vi "Dashboard Main.vi"() -> ()   [LabVIEW 2017]
uses:
  RoboRio Code/Systems/Autonomous/Autonomous/ENUM_Auto_AutoMode.ctl
  RoboRio Code/Systems/Arm/ENUM_SM_State.ctl
  RoboRio Code/Systems/Claw Rotation/ENUM_SM_State.ctl
  RoboRio Code/Systems/Lift/ENUM_SM_State.ctl
  <vilib>/Utility/miscctls.llb/LVRowAndColumnTypeDef.ctl
  <vilib>/event_ctls.llb/eventvkey.ctl
  RoboRio Code/TypeDef/CLUSTER_Sensitivities.ctl
  <vilib>/Rock Robotics/Network Tables/NT Read Numeric Array.vi
  <vilib>/Rock Robotics/WPI/Dashboard/WPI_DashboardLogging Global.vi
  RoboRio Code/Systems/Arm/Arm.lvlib
  RoboRio Code/Systems/Claw Rotation/Claw_Rotation.lvlib
  RoboRio Code/Systems/Lift/Lift.lvlib
panel:
  in  "Camera Settings Right":T1={"Frame Rate"=30, "Compression"=30, "Size"=1, "DB Camera Config"=FALSE} {"Frame Rate" scale=1.0..30.0; "Compression" scale=100.0..-1.0; "Size" items=["640x480", "320x240", "160x120"]}
  in  "Camera Name Right":string(combo)="No Camera Selection"
  out "Camera Info":cluster{"Mbps LED":bool, "Mbps":dbl, "fps":dbl} {"fps" format="%#.1g"; "Mbps" format="%#.1g"}
  in  "Camera Settings":T1={"Frame Rate"=30, "Compression"=30, "Size"=1, "DB Camera Config"=FALSE} {"Frame Rate" scale=1.0..30.0; "Compression" scale=100.0..-1.0; "Size" items=["640x480", "320x240", "160x120"]}
  in  "TCP":refnum<k5>
  in  "Rec Mode":enum32{"Stop", "Record", "Playback"}(radio)
  out "Robot IP":string
  out "Image Message":string="Timeout in Camera Communications"
  in  "Dashboard Tab":T2(tab)
  in  "Select Auto":string(combo)="Select Autonomous ..."
  out "NT Connection":bool
  out "MotorChart R":cluster{"Numeric":dbl, "Numeric":dbl}(graph)
  out "MotorChart L":cluster{"Numeric":dbl, "Numeric":dbl}(graph)
  out "MotorSliders R":cluster{"MotorSlide1":dbl, "MotorSlide2":dbl} {"MotorSlide2" scale=-1.0..1.0 scale format="%#_2e"; "MotorSlide1" scale=-1.0..1.0 scale format="%#_2e"}
  out "MotorSliders L":cluster{"MotorSlide1":dbl, "MotorSlide2":dbl} {"MotorSlide2" scale=-1.0..1.0 scale format="%#_2e"; "MotorSlide1" scale=-1.0..1.0 scale format="%#_2e"}
  out "Gyro":dbl(knob) scale=0.0..360.0
  out "JS1 Z":dbl(slide) scale=-1.0..1.0 scale format="%#_2e"
  out "JS1 Graph":cluster{"X":dbl, "Y":dbl}[](graph)
  out "JS1 Buttons":T3
  out "JS2 Z":dbl(slide) scale=-1.0..1.0 scale format="%#_2e"
  out "JS2 Graph":cluster{"X":dbl, "Y":dbl}[](graph)
  out "JS2 Buttons":T3
  out "Mode":T4(ring)=enum."Auto Disabled"
  out "Camera Image Right":T5(plugin-control)
  out "Lift State":T6
  out "Claw Rotation State":T7
  out "Arm State":T8
  in  "Low Gear Sen Min":dbl
  in  "Low Gear Sen Max":dbl
  in  "High Gear Sen Min":dbl
  in  "High Gear Sen Max":dbl
  out "Bottom Arm":bool
  out "Top Arm":bool
  out "Bottom Claw":bool
  out "Top Claw":bool
  out "Bottom Lift":bool
  out "Top Lift":bool
  out "Cube":bool
  out "Road Nav":bool
  out "Cube":bool
  out "Low Gear":bool
  out "High Gear":bool
  out "Drive Mode":T9(ring)
  out "Lock Angle":bool
  out "Turbo Enabled":bool
  out "Comp. Running":bool
  out "Comp. Enabled":bool
  in  "Reset Max RPM":bool
  out "Right Max":dbl
  out "Left Max":dbl
  out "Right":dbl
  out "Left":dbl
  out "Battery Meter":dbl(knob) scale=0.0..15.0
  in  "Cube Steer Scale":dbl
  in  "Cube Deadband":dbl
  in  "Auto Route":T10
  out "V Min":dbl
  out "V Max":dbl
  in  "V Values":cluster{dbl, dbl}(slide) scale=0.0..255.0
  out "S Min":dbl
  out "S Max":dbl
  in  "S Values":cluster{dbl, dbl}(slide) scale=0.0..255.0
  out "H Min":dbl
  out "H Max":dbl
  in  "H Values":cluster{dbl, dbl}(slide) scale=0.0..255.0
  in  "Test Slider":dbl(slide) scale=0.0..100.0 scale format="%#_3g"
  in  "On/Off":bool caption="Solenoid"
  in  "Test Name":u16(ring) items=["Select the test to run..."]
  in  "Test Tree":string(tree)
  in  "Motor":cluster{"Value":dbl, "Enable":bool} {"Value" scale=-1.0..1.0 scale format="%#_3g"}
  out "Progress":T11 {"Test Progress" scale=0.0..100.0}
  in  "Rev/Fwd":cluster{"Forward":bool, "Reverse":bool}
  in  "Test Ring":u16(ring) items=["Monochrome", "Color"]
  out "Cmd Status":string
  in  "Execute Command":bool
  in  "Command Params":string[][](table)
  in  "Command Selection":i32(listbox)
  in  "CheckList":i32(listbox)
  out "Tree":string(tree)
  out "Manipulator Mietus":picture
  out "Handsome Hale":picture
  out "Jeffery Junior":picture
  out "Camera Image":T5(plugin-control)
  in  "Camera Name":string(combo)="No Camera Selection"
  # "HW"
  # "HW"
  # "Joysticks"
  # "Drive Motors"
  # "Front"
  # "Right"
  # "Left"
  # "Back"
  # "Drive RPMs"
  # "Limit Switches"
  # "Drive"
  # "Object Tracker"
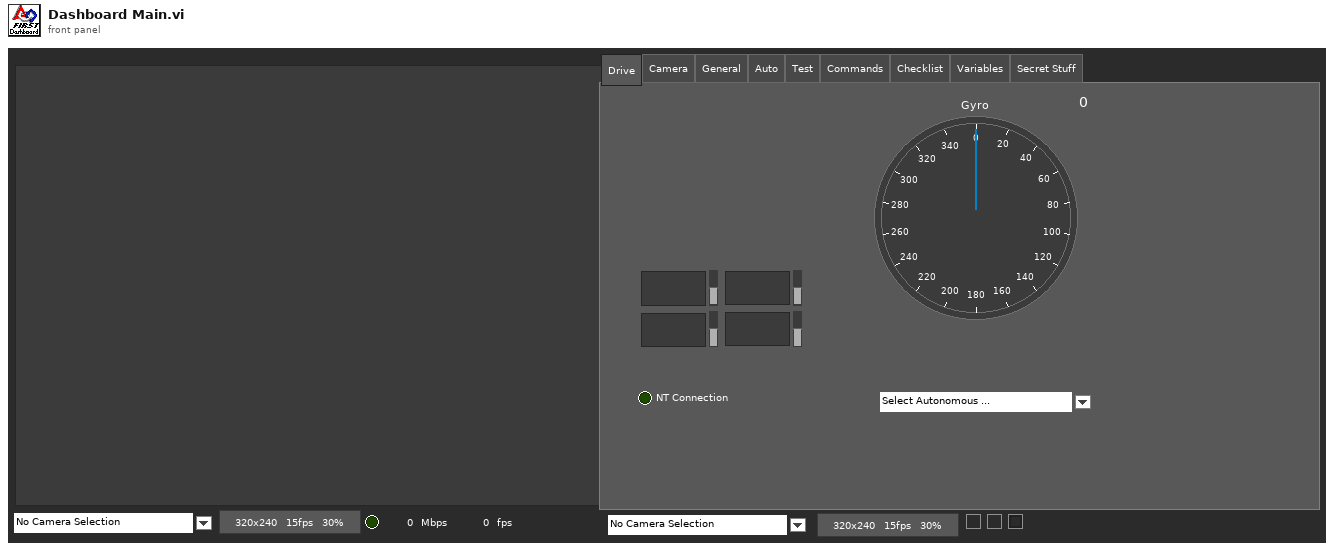
[diagram p1: front panel]
types:
  T1 = cluster{"Frame Rate":i32, "Compression":i32, "Size":u16, "DB Camera Config":bool}
  T2 = enum32{"Drive", "Camera", "General", "Auto", "Test", "Commands", "Checklist", "Variables", "Secret Stuff"}
  T3 = cluster{bool, bool, bool, bool, bool, bool, bool, bool, bool, bool, bool, bool}
  T4 = enum8{"Tele-Op Disabled", "Tele-Op Enabled", "Auto Disabled", "Auto Enabled", "Test Disabled", "Test Enabled", "Disconnected", "No Code", "E-Stop"}
  T5 = typedef "IMAQ Image.ctl" = refnum<image>
  T6 = typedef "Lift.lvlib/ENUM_SM_State.ctl" = enum16{"Startup", "Idle", "F_Manual", "Manual", "Position - Moving", "Position - Holding", "Shutdown"}
  T7 = typedef "Claw_Rotation.lvlib/ENUM_SM_State.ctl" = enum16{"Startup", "Idle", "F_Manual", "Manual", "Position - Moving", "Position - Holding", "Shutdown"}
  T8 = typedef "Arm.lvlib/ENUM_SM_State.ctl" = enum16{"Startup", "Idle", "F_Manual", "Manual", "Position - Moving", "Position - Holding", "Shutdown"}
  T9 = enum16{"Motion Profile", "CrossLineAuto", "VBus", "Stop"}
  T10 = typedef "ENUM_Auto_AutoMode.ctl" = enum16{"No Movement", "Scale And Switch", "Switch", "Scale", "Cross Line"}
  T11 = cluster{"Test Progress":u8, "Test Progress Text":string}
  T12 = cluster{"Save Path":path, "Interval (s)":dbl, "Keep":i32}
  T13 = enum32{"General", "Drive", "Camera", "Basic", "Custom", "Test", "Commands", "Checklist", "Variables"}
  T14 = typedef "Image Type" = u32
  T15 = cluster{"IDs":cluster{"RPC field ID":u16, "Unique ID":u16}, "String":string}
  T16 = enum32{"Drive", "Camera", "General", "Auto", "Test", "Commands", "Checklist", "Variables"}
  T17 = cluster{"Camera Image":refnum<vi>, "Dashboard Tab":refnum<vi>, void, "Rec Mode":refnum<vi>, "Test Slider":refnum<vi>, "On/Off ":refnum<vi>, "Test Ring":refnum<vi>, "Rev/Fwd":refnum<vi>, "Test Name":refnum<vi>, "Motor":refnum<vi>, "Progress":refnum<vi>, "CheckList":refnum<vi>, "Tree":refnum<vi>, "Test Tree":refnum<vi>, "Command Params":refnum<vi>, "Command Selection":refnum<vi>, "Execute Command":refnum<vi>, "Cmd Status":refnum<vi>, "Camera Settings":refnum<vi>, "Camera Name":refnum<vi>, "Camera Info":refnum<vi>, "Camera Settings Right":refnum<vi>, "Camera Name Right":refnum<vi>, "Camera Image Right":refnum<vi>}
  T18 = cluster{"Camera Name":string, string, "Saved DB Images Info":cluster{"Save Path":path, "Interval (s)":dbl, "Keep":i32}}
  T19 = cluster{"Camera Name Right":string, string, "Saved DB Images Info":cluster{"Save Path":path, "Interval (s)":dbl, "Keep":i32}}
  T20 = typedef "CLUSTER_Sensitivities.ctl" = cluster{"High Gear Max":dbl, "High Gear Min":dbl, "Low Gear Max":dbl, "Low Gear Min":dbl}
  T21 = cluster{"Error Strings":string, "Disable Counts":cluster{u16, u16}, "Rail Faults":cluster{u16, u16, u16}, "Robot IP":string, "DB Mode":u8, "Event Info":cluster{"Name":string, "Type":u8, "Number":u16, "Replay":u8}}
  T22 = cluster{"Storage":cluster{"Disk Free":u64, "RAM Block":u32, "RAM free":u32}, "CPU Utilization":cluster{"CPU % ISR":sgl, "CPU % Time Crit":sgl, "CPU % Timed Str":sgl, "CPU % High":sgl, "CPU % Above":sgl, "CPU % Normal":sgl, "CPU % Low":sgl}, "CAN":cluster{"% Bus Utilization":sgl, "Bus Off Cnt":u32, "TX_FIFO Full Cnt":u32, "Receive Error Cnt":u8, "Transmit Error Cnt":u8}, "HID":cluster{"HID Outputs":u32, "Rumble Low":u16, "Rumble High":u16}[]}
  T23 = cluster{"Status bits":cluster{"Test Mode":bool, "Autonomous":bool, "Enabled":bool, "Code Start":bool, "Brownout":bool, "Reserved 2":bool, "Reserved 3":bool, "E-Stop":bool}, "Code Trace":cluster{"Disabled":bool, "TeleOp":bool, "Auto":bool, "Test":bool}, "Controller Type":enum16{"unknown", "cRIO", "roboRio"}, "Code?":enum16{"unknown", "noCode", "code"}, "Battery V":dbl}
  T24 = cluster{"Control Bits":cluster{"TestMode":bool, "Autonomous":bool, "Enabled":bool, "FMS Present":bool, bool, bool, bool, "E-Stop":bool}, "Team Station ":u8, "Countdown":sgl, "Joystick Values":cluster{"Axes":dbl[], "Buttons":bool[], "POVs":i16[]}[]}
  T25 = cluster{"Axes":dbl[], "Buttons":bool[], "POVs":i16[]}[]
  T26 = typedef "Cluster_Compressor.ctl" = cluster{"Compressor Running":bool, "Compressor Enabled":bool}
  T27 = typedef "CLUSTER_CMD_WC_Drive.ctl" = cluster{"Drive_Mode":T28, "VBus":T29, "Profile":T31, "Zero Drive Encoders":bool, "Set Target Position(IN)":dbl, "Target Angle(Degree)":dbl, "Lock Angle":bool, "Zero YAW":bool, "Follow Cubes":bool, "Follow Road":bool}
  T28 = typedef "ENUM_WC_Drive_DriveMode.ctl" = enum16{"Motion Profile", "CrossLineAuto", "VBus", "Stop"}
  T29 = typedef "CLUSTER_Drive_ACT Loop_VBus Data.ctl" = cluster{"Drive":T30, "Turbo":bool}
  T30 = typedef "CLUSTER_X and Y.ctl" = cluster{"Steer":dbl, "Throtle":dbl}
  T31 = typedef "CLUSTER_Drive_ACT Loop_Profile Data.ctl" = cluster{"Start":bool}
  T32 = cluster{"Axes":dbl[], "Buttons":bool[], "POVs":i16[]}
  T33 = cluster{"Buttons[0]":bool, "Buttons[1]":bool, "Buttons[2]":bool, "Buttons[3]":bool, "Buttons[4]":bool, "Buttons[5]":bool, "Buttons[6]":bool, "Buttons[7]":bool, "Buttons[8]":bool, "Buttons[9]":bool, "Buttons[10]":bool, "Buttons[11]":bool}
  T34 = typedef "CLUSTER_Limit_Switches.ctl" = cluster{"Cube":bool, "Top Arm":bool, "Bottom Claw":bool, "Top Lift":bool, "Bottom Arm":bool, "Bottom Lift":bool, "Top Claw":bool}
  T35 = cluster{"Operation":enum16{"Update", "Clear"}, "Color Box":u32}[]
  T36 = typedef "eventvkey.ctl" = enum16{"ASCII", "Enter", "Return", "Shift", "Ctrl", "Alt", "Cmd", "Opt", "Caps", "NumLock", "Clear", "Break", "Up", "Down", "Left", "Right", "Insert", "Delete", "Home", "End", "PageUp", "PageDown", "Escape", "Help", "Pause", "ScrollLock", "F1", "F2", "F3", "F4", "F5", "F6", "F7", "F8", "F9", "F10", "F11", "F12", "F13", "F14", "F15", "F16", "F17", "F18", "F19", "F20", "F21", "F22", "F23", "F24", "Play", "VolumeUp", "VolumeDown", "Mute", "Two Byte Char"}
  T37 = cluster{"Image Size":bool, "Image Type":bool, "Pixel Value":bool, "ROI Information":bool, "Zoom Factor":bool}
  T38 = cluster{"Operation":enum16{"Update", "Clear"}, "Color Box":u32}
  T39 = typedef "LVRowAndColumnTypeDef.ctl" = cluster{"Row":i32, "Column":i32}
  T40 = cluster{"Shift":bool, "Ctrl":bool, "Alt":bool, "Cmd":bool, "Opt":bool}
  T41 = typedef "imagedata.ctl" = cluster{"image type":i32, "image depth":i32, "image":u8[], "mask":u8[], "colors":u32[], "Rectangle":cluster{"left":i16, "top":i16, "right":i16, "bottom":i16}}
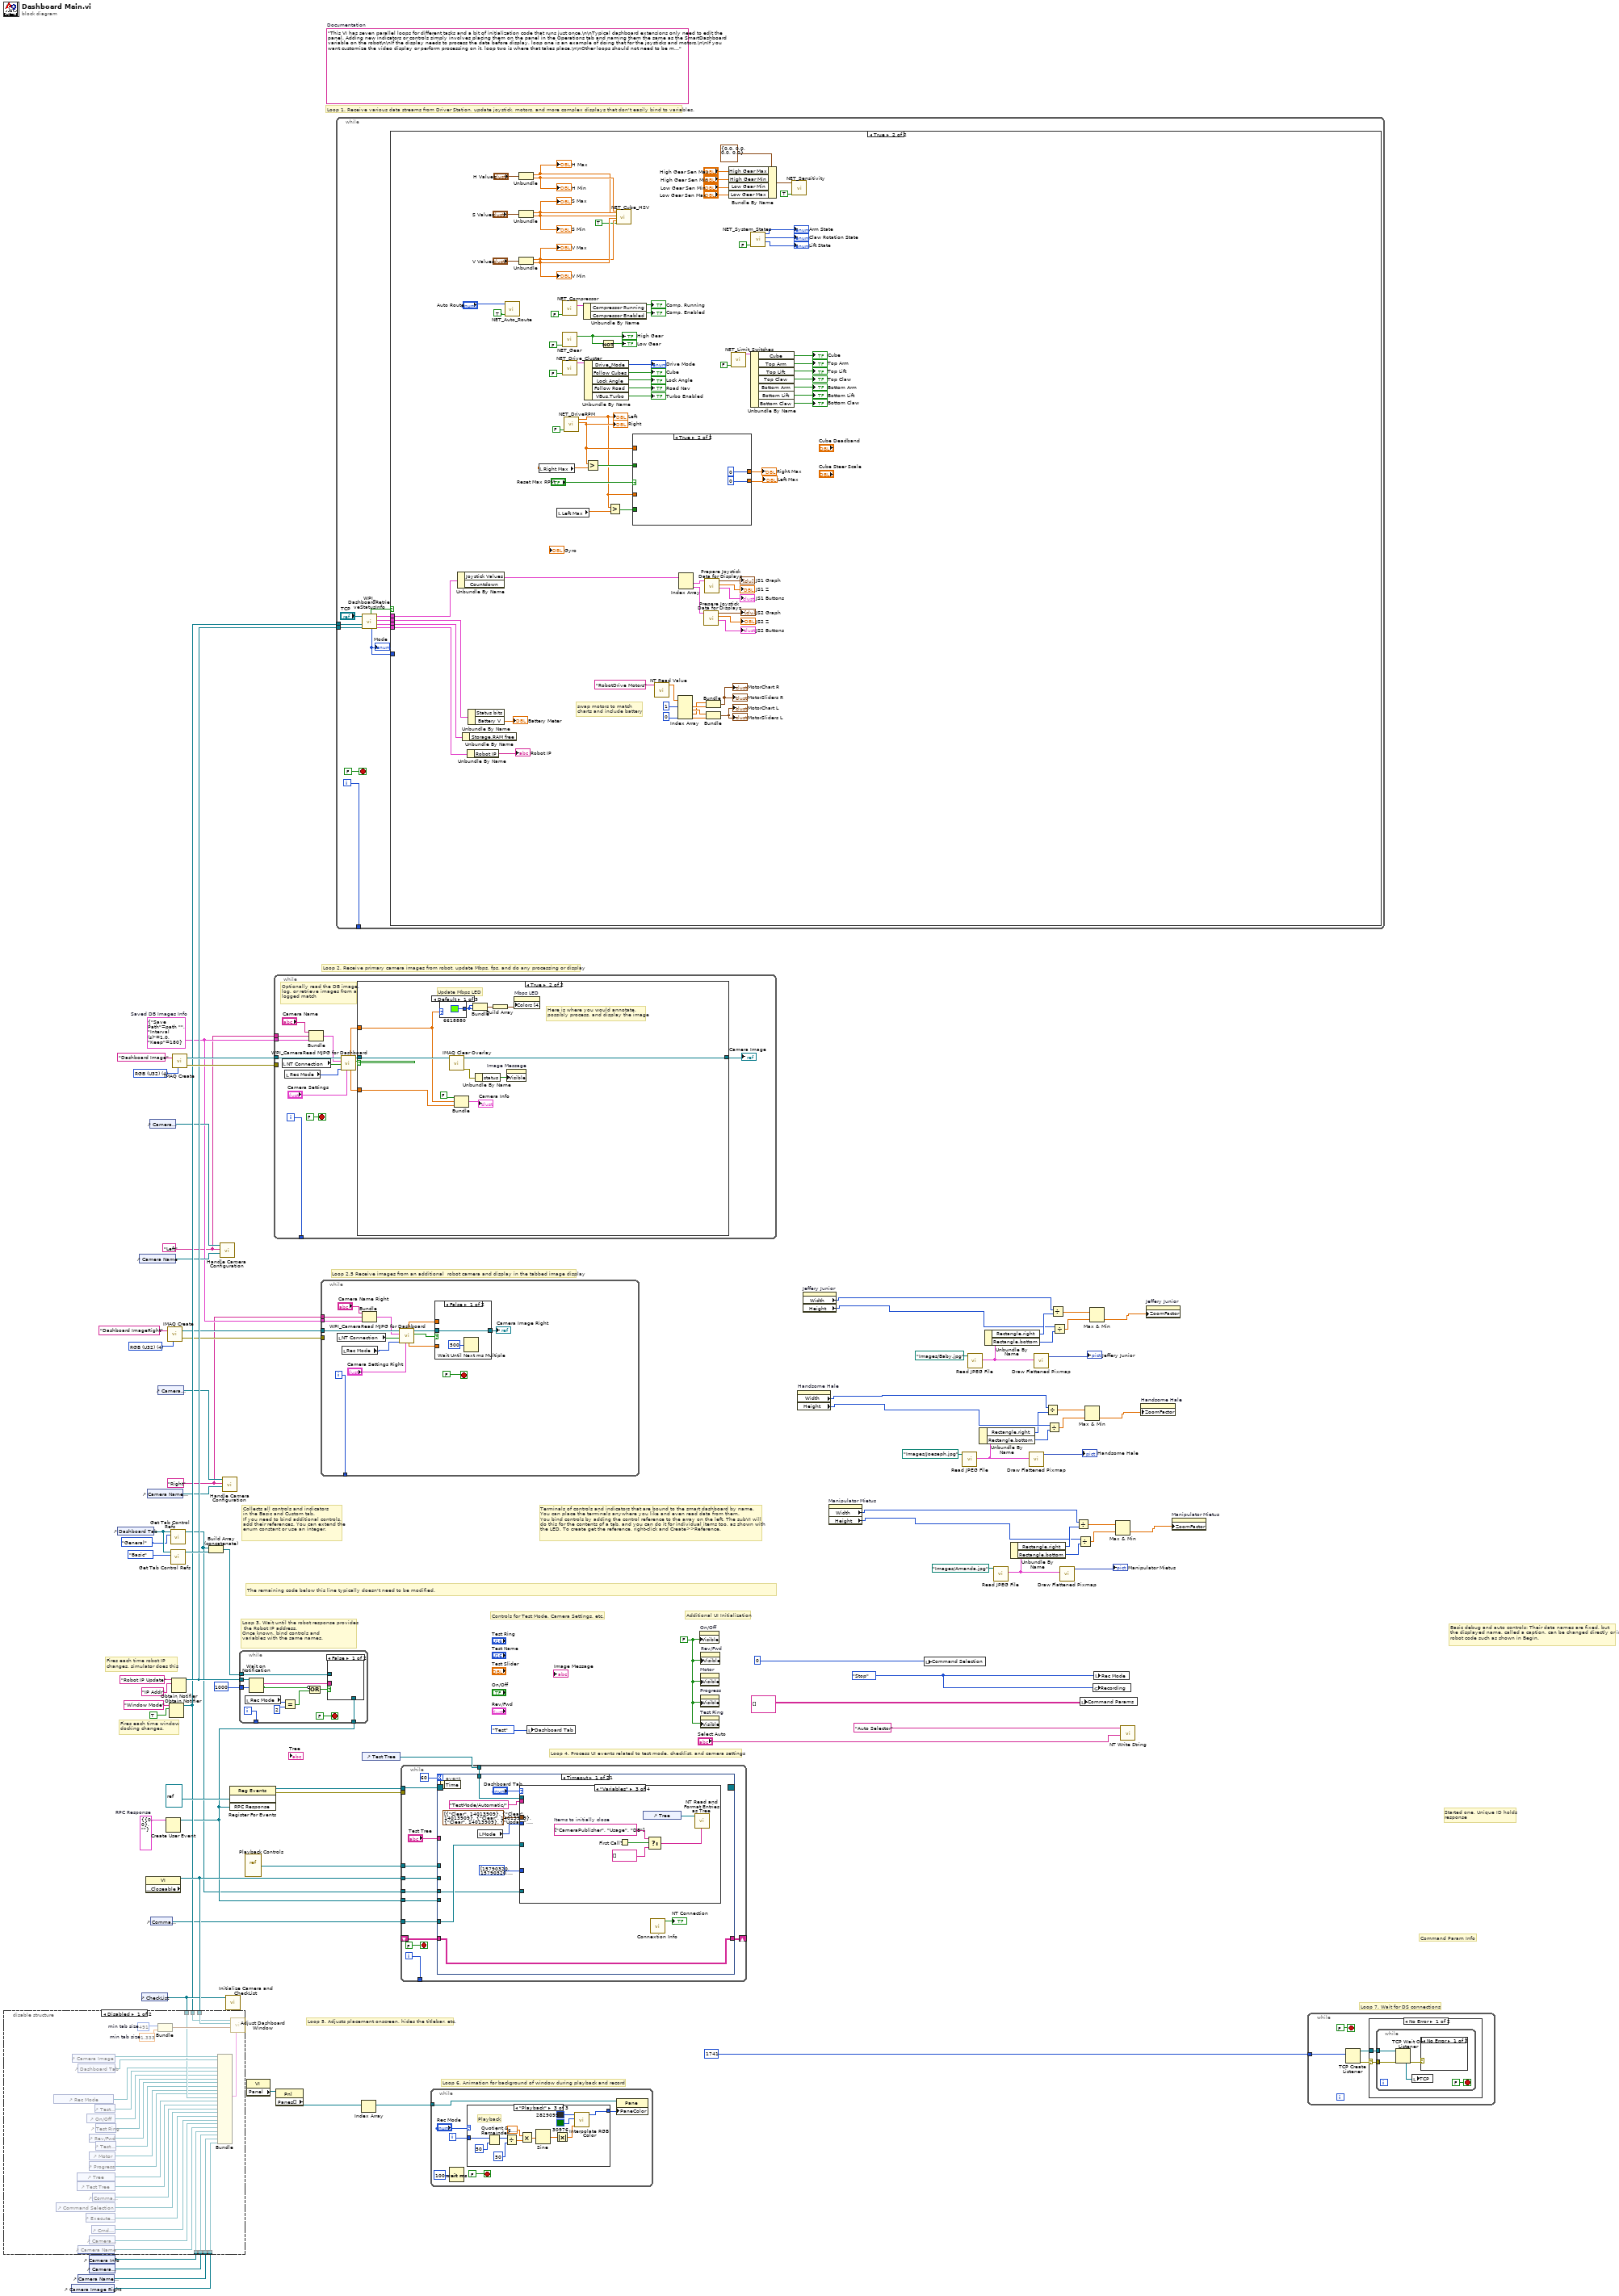
[diagram p0: block diagram]
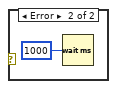
[diagram p4: hidden frame]
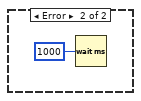
[diagram p5: hidden frame]
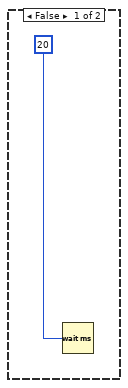
[diagram p6: hidden frame]
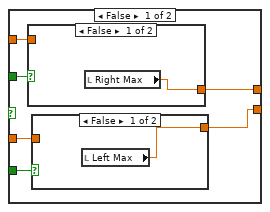
[diagram p7: hidden frame]
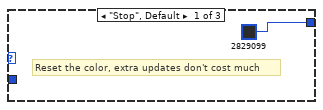
[diagram p10: hidden frame]
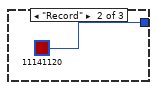
[diagram p11: hidden frame]
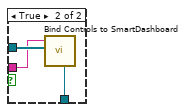
[diagram p12: hidden frame]
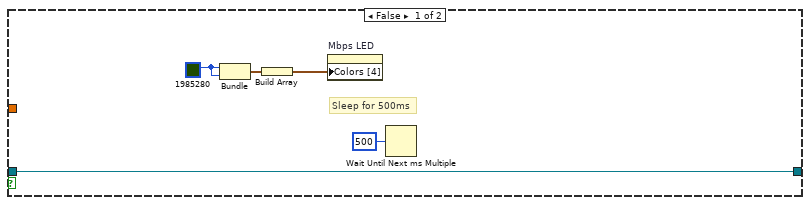
[diagram p13: hidden frame]
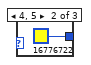
[diagram p14: hidden frame]
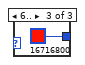
[diagram p15: hidden frame]
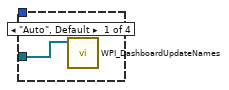
[diagram p16: hidden frame]
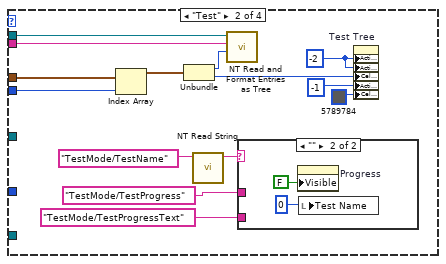
[diagram p17: hidden frame]
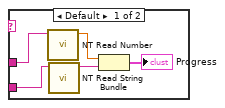
[diagram p18: hidden frame]
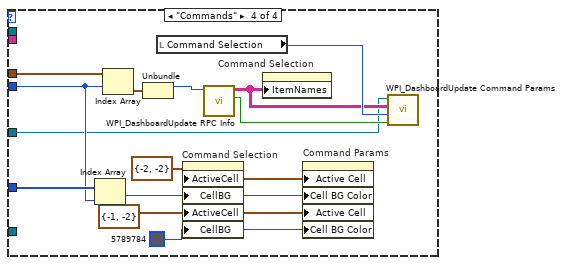
[diagram p19: hidden frame]
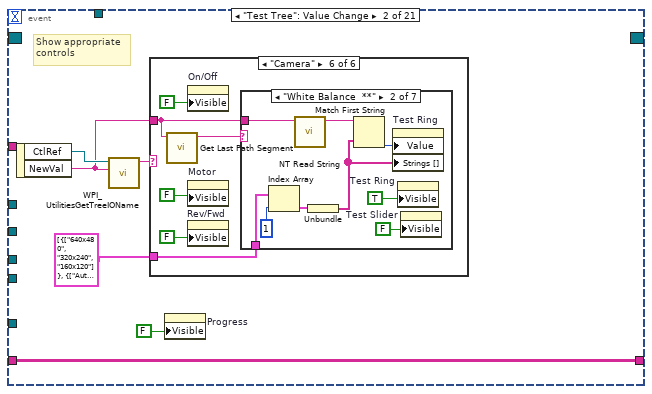
[diagram p20: hidden frame]
diagram:
  w34 = T12 {"Save Path"=path "", "Interval (s)"=1.0, "Keep"=180}  # Saved DB Images Info
  w33 = "Right"
  w32 = "Left"
  w44 = T14 4 items=["Grayscale (U8)", "Grayscale (I16)", "Grayscale (SGL)", "Complex (CSG)", "RGB (U32)", "HSL (U32)", "RGB (U64)"] ("Image Type")
  w55 = T15 {"IDs"={"RPC field ID"=0, "Unique ID"=0}, "String"=""}  # RPC Response
  w66 = enum32{"Stop", "Record", "Playback"}."Stop" ("Rec Mode")
  w60 = FALSE ("Visible")
  (unwired) "This VI has seven parallel loops for different tasks and a bit of initialization code that runs just once.\n\nTypical dashboard extensions only need to edit the panel. Adding new indicators or controls simply involves placing them on the panel in the Operations tab and naming them the same as the SmartDashboard variable on the robot\n\nIf the display needs to process the data before display, loop one is an example of doing that for the joysticks and motors.\n\nIf you want customize the video display or perform processing on it, loop two is where that takes place.\n\nOther loops should not need to be modified. They are pretty standard, and document the task they perform."  # Documentation
  w83 = T14 4 items=["Grayscale (U8)", "Grayscale (I16)", "Grayscale (SGL)", "Complex (CSG)", "RGB (U32)", "HSL (U32)", "RGB (U64)"] ("Image Type")
  # "Loop 2.5 Receive images from an additional  robot camera and display in the tabbed image display"
  # "Command Param Info"
  # "Started one, Unique ID holds\nresponse"
  # "Loop 7. Wait for DS connections"
  # "Basic debug and auto controls: Their data names are fixed, but\nthe displayed name, called a caption, can be changed directly or in\nrobot code such as shown in Begin."
  # "Controls for Test Mode, Camera Settings, etc."
  # "Additional UI Initialization"
  # "Loop 6. Animation for background of window during playback and record"
  # "Fires each time robot IP\nchanges, simulator does this"
  # "Fires each time window\ndocking changes."
  # "Collects all controls and indicators\nin the Basic and Custom tab.\nIf you need to bind additional controls,\nadd their references. You can extend the\nenum constant or use an integer."
  # "The remaining code below this line typically doesn't need to be modified."
  # "Loop 4. Process UI events related to test mode, checklist, and camera settings"
  # "Terminals of controls and indicators that are bound to the smart dashboard by name.\nYou can place the terminals anywhere you like and even read data from them.\nYou bind controls by adding the control reference to the array on the left. The subVI will\ndo this for the contents of a tab, and you can do it for individual items too, as shown with\nthe LED. To create get the reference, right-click and Create>>Reference."
  # "Loop 3. Wait until the robot response provides\n the Robot IP address.\nOnce known, bind controls and\nvariables with the same names."
  # "Loop 5. Adjusts placement onscreen, hides the titlebar, etc."
  # "Loop 1. Receive various data streams from Driver Station, update joystick, motors, and more complex displays that don't easily bind to variables."
  # "Loop 2. Receive primary camera images from robot, update Mbps, fps, and do any processing or display"
  n1 = control-ref of="Camera Image Right"() -> (w37:refnum<vi>)
  n2 = control-ref of="Camera Name Right"() -> (w38:refnum<vi>)
  n3 = control-ref of="Camera Info"() -> (w49:refnum<vi>)
  n4 = control-ref of="Camera Settings Right"() -> (w39:refnum<vi>)
  n5 = control-ref of="Dashboard Tab"() -> (w64:refnum<vi>)
  n6 = control-ref of="Camera Name"() -> (w50:refnum<vi>)
  n7 = control-ref of="CheckList"() -> (w61:refnum<vi>)
  n8 = property class="VI" props=["Front Panel.Closeable"]() -> (reference out=w65:refnum<vi>)  [unwired: 2 in, 2 out]
  n9 = control-ref of="Camera Name Right"() -> (w40:refnum<vi>)
  n10 = control-ref of="Camera Settings"() -> (w51:refnum<vi>)
  n11 = control-ref of="Command Params"() -> (w52:refnum<vi>)
  n12 = control-ref of="Camera Settings Right"() -> (w41:refnum<vi>)
  n13 = Create User Event(user event datatype=w55) -> (user event=w53:refnum<user-event>)  [unwired: 1 in, 1 out]
  n14 = call "IMAQ Create"("Image Name"="Dashboard ImageRight", "Image Type"=w44) -> ("New Image"=w43:T5, "error out"=w42:errorcluster)  [unwired: 2 in, 1 out]
  n15 = Obtain Notifier(name (unnamed)="Window Mode", notification data type=TRUE) -> (notifier out=w58:refnum<notifier>)  [unwired: 2 in, 2 out]
  n16 = disable-structure shown="Disabled" {
    disable-tunnel: w65 -> [w113 _]
    disable-tunnel: w61 -> [w105 _]
    disable-tunnel: w58 -> [w94 _]
    disable-tunnel: w49 -> [w87 _]
    disable-tunnel: w39 -> [w86 _]
    disable-tunnel: w38 -> [w85 _]
    disable-tunnel: w37 -> [w84 _]
    frame Disabled {
      w110 = 491  # min tab size
      w109 = 1.333  # min tab size
      n17 = control-ref of="Rec Mode"() -> (w100:refnum<vi>)
      n18 = control-ref of="Command Selection"() -> (w91:refnum<vi>)
      n19 = control-ref of="Camera Image"() -> (w112:refnum<vi>)
      n20 = control-ref of="Tree"() -> (w104:refnum<vi>)
      n21 = control-ref of="Test Tree"() -> (w103:refnum<vi>)
      n22 = control-ref of="Dashboard Tab"() -> (w111:refnum<vi>)
      n23 = control-ref of="Camera Name"() -> (w88:refnum<vi>)
      n24 = control-ref of="Execute Command"() -> (w92:refnum<vi>)
      n25 = control-ref of="On/Off"() -> (w98:refnum<vi>)
      n26 = control-ref of="Progress"() -> (w95:refnum<vi>)
      n27 = control-ref of="Camera Settings"() -> (w89:refnum<vi>)
      n28 = control-ref of="Rev/Fwd"() -> (w96:refnum<vi>)
      n29 = control-ref of="Motor"() -> (w101:refnum<vi>)
      n30 = control-ref of="Cmd Status"() -> (w90:refnum<vi>)
      n31 = control-ref of="Command Params"() -> (w93:refnum<vi>)
      n32 = control-ref of="Test Slider"() -> (w99:refnum<vi>)
      n33 = control-ref of="Test Ring"() -> (w97:refnum<vi>)
      n34 = control-ref of="Test Name"() -> (w102:refnum<vi>)
      n35 = Bundle("min tab size"=w110, "min tab size"=w109) -> (w108:cluster{"min tab size":i32, "min tab size":dbl})  [unwired: 1 in]
      n36 = Bundle("Camera Image"=w112, "Dashboard Tab"=w111, "Rec Mode"=w100, "Test Slider"=w99, "On/Off"=w98, "Test Ring"=w97, "Rev/Fwd"=w96, "Test Name"=w102, "Motor"=w101, "Progress"=w95, "CheckList"=w105, "Tree"=w104, "Test Tree"=w103, "Command Params"=w93, "Command Selection"=w91, "Execute Command"=w92, "Cmd Status"=w90, "Camera Settings"=w89, "Camera Name"=w88, "Camera Info"=w87, "Camera Settings Right"=w86, "Camera Name Right"=w85, "Camera Image Right"=w84) -> (w106:T17, w107)  [unwired: 1 in]
      n37 = call "Adjust Dashboard Window.vi"("Sizing Refnums"=w106, "Size Constraints"=w108, "VI"=w113, "WIn Mode"=w94) -> ()  [unwired: 8 in]
    }
    frame Enabled {
    }
  }
  n38 = call <vilib>:"Get Tab Control Refs.vi"("Page Index"=T13."General" ("Dashboard Tab"), "TabControl in"=w64) -> ("ControlsOnPage"=w48:refnum<vi>[])  [unwired: 9 in]
  n39 = call <vilib>:"Get Tab Control Refs.vi"("Page Index"=T13."Basic" ("Dashboard Tab"), "TabControl in"=w64) -> ("ControlsOnPage"=w63:refnum<vi>[])  [unwired: 9 in]
  n40 = Obtain Notifier(name (unnamed)="Robot IP Update", notification data type="IP Addr" ("name (unnamed)")) -> (notifier out=w59:refnum<notifier>)  [unwired: 2 in, 2 out]
  n41 = call "IMAQ Create"("Image Name"="Dashboard Image", "Image Type"=w83) -> ("New Image"=w81:T5, "error out"=w80:errorcluster)  [unwired: 2 in, 1 out]
  n42 = Build Array (concatenate)(w48, w63) -> (w62:refnum<vi>[])
  n43 = call "Handle Camera Configuration.vi"("CameraNameRef"=w50, "Display Name"=w32, "ClusterRef"=w51) -> ()  [unwired: 9 in]
  n44 = call "Handle Camera Configuration.vi"("CameraNameRef"=w40, "Display Name"=w33, "ClusterRef"=w41) -> ()  [unwired: 9 in]
  n45 = call "Initialize Camera and CheckList.vi"("ListBox in"=w61) -> ()  [unwired: 11 in]
  n46 = register-events(refnum<vi> refnum, w53) -> (reference out=w70:refnum<event-registration>, error out=w69:errorcluster)  [unwired: 2 in]
  n47 = while {
    tunnel: w62 -> [w125]
    tunnel: w59 -> [w123]
    tunnel: [w121] -> _
    tunnel: u32 1000 ("milliseconds to wait") -> [w120]
    tunnel: w53 -> [w114]
    i -> [w121]
    stop <- FALSE stop-if-true
    n48 = local read "Rec Mode"() -> (w116:enum32{"Stop", "Record", "Playback"})
    n49 = Wait on Notification(notifier=w123, timeout in ms (-1)=w120) -> (notification=w122:string, timed out?=w118:bool)  [unwired: 2 in, 2 out]
    n50 = Equal?(x=w116, y=u16 2 ("Rec Mode")) -> (x = y?=w117:bool)
    n51 = Compound Arithmetic op=OR(invert w118, w117) -> (w119:bool)
    n52 = case shown="False" w119 {
      tunnel: w125 -> [_ w128]
      tunnel: w122 -> [_ w127]
      tunnel: w114 -> [_ w126]
      frame False {
      }
      frame True {
        n53 = call <vilib>:"Bind Controls to SmartDashboard.vi"("RPC ref"=w126, "Bound Control Refs"=w128, "Server IP Address"=w127) -> ()  [unwired: 9 in]
      }
    }
  }
  n54 = vi-ref "Playback Controls.vi"() -> (w71:refnum<vi>)
  n55 = property class="VI"() -> ("Panel"=w73:refnum<vi>)  [unwired: 2 in, 2 out]
  n56 = while {
    tunnel: w81 -> [w141]
    tunnel: w80 -> [_]
    tunnel: [w142] -> _
    tunnel: w34 -> [w132]
    tunnel: w32 -> [w129]
    i -> [w142]
    stop <- FALSE stop-if-true
    # "Optionally read the DB image,\nlog, or retrieve images from a\nlogged match"
    n57 = local read "NT Connection"() -> (w133:bool)
    n58 = local read "Rec Mode"() -> (w137:enum32{"Stop", "Record", "Playback"})
    n59 = Bundle("Camera Name"="Camera Name", w129, "Saved DB Images Info"=w132) -> (w131:T18)  [unwired: 1 in]
    n60 = call <vilib>:"WPI_CameraRead MJPG for Dashboard.vi"("Camera Settings"="Camera Settings", "Rec Mode"=w137, "NT Connection"=w133, "Capture Info"=w131, "Refnum in"=w141) -> ("Active"=w139:bool, "Refnum out"=w140:T5, "FPS"=w138:dbl, "Bandwidth (Mbps)"=w136:dbl)  [unwired: 3 in]
    n61 = case shown="True" w139 {
      tunnel: w140 -> [w144 w155]
      tunnel: w136 -> [_ w152]
      tunnel: w138 -> [_ w153]
      tunnel: [w144 w149] -> w134
      frame False {
        w146 = u32 1985280 ("Color Box")
        # "Sleep for 500ms"
        n62 = Bundle("Color Box"=w146, "Color Box"=w146) -> (w147:cluster{"Color Box":u32, "Color Box":u32})  [unwired: 1 out]
        n63 = Build Array(w147) -> (w145:cluster{"Color Box":u32, "Color Box":u32}[])
        n64 = property on="Mbps LED" class="Bool (strict)"("Colors [4]"=w145) -> ()  [unwired: 2 in, 2 out]
        n65 = Wait Until Next ms Multiple(millisecond multiple=u32 500) -> ()  [unwired: 1 out]
      }
      frame True {
        # "Here is where you would annotate,\npossibly process, and display the image"
        # "Update Mbps LED"
        n66 = case shown="Default" w152 {
          tunnel: [u32 6618880 ("Color Box") u32 16776722 ("Color Box") u32 16716800 ("Color Box")] -> w156
          frame Default {
          }
          frame 4, 5 {
          }
          frame 6.. {
          }
        }
        n67 = call "IMAQ Clear Overlay"("Image"=w155) -> ("error out"=w158:errorcluster, "Image Out"=w149:T5)  [unwired: 2 in, 7 out]
        n68 = Bundle(FALSE, "Bandwidth (Mbps)"=w152, "FPS"=w153) -> (→"Camera Info":cluster{bool, "Bandwidth (Mbps)":dbl, "FPS":dbl})  [unwired: 1 in]
        n69 = Bundle("Color Box"=w156, "Color Box"=w156) -> (w157:cluster{"Color Box":u32, "Color Box":u32})  [unwired: 1 out]
        n70 = Unbundle By Name(w158) -> ("status"=w159:bool)
        n71 = Build Array(w157) -> (w154:cluster{"Color Box":u32, "Color Box":u32}[])
        n72 = property on="Image Message" class="Str"("Visible"=w159) -> ()  [unwired: 2 in, 2 out]
        n73 = property on="Mbps LED" class="Bool (strict)"("Colors [4]"=w154) -> ()  [unwired: 2 in, 2 out]
      }
    }
    "Camera Image" <- w134
  }
  n74 = property class="Pnl"(reference=w73) -> ("Panes[]"=w74:refnum<vi>[])  [unwired: 1 in, 2 out]
  n75 = while {
    tunnel: w43 -> [w177]
    tunnel: w42 -> [_]
    tunnel: [w172] -> _
    tunnel: w34 -> [w166]
    tunnel: w33 -> [w163]
    i -> [w172]
    stop <- FALSE stop-if-true
    n76 = local read "NT Connection"() -> (w167:bool)
    n77 = local read "Rec Mode"() -> (w176:enum32{"Stop", "Record", "Playback"})
    n78 = Bundle("Camera Name Right"="Camera Name Right", w163, "Saved DB Images Info"=w166) -> (w165:T19)  [unwired: 1 in]
    n79 = call <vilib>:"WPI_CameraRead MJPG for Dashboard.vi"("Camera Settings"="Camera Settings Right", "Rec Mode"=w176, "NT Connection"=w167, "Capture Info"=w165, "Refnum in"=w177) -> ("Active"=w171:bool, "Refnum out"=w174:T5, "FPS"=w169:dbl, "Bandwidth (Mbps)"=w170:dbl)  [unwired: 3 in]
    n80 = case shown="False" w171 {
      tunnel: w174 -> [w178 w180]
      tunnel: w170 -> [_ _]
      tunnel: w169 -> [_ _]
      tunnel: [w178 w180] -> w168
      frame False {
        n81 = Wait Until Next ms Multiple(millisecond multiple=u32 500) -> ()  [unwired: 1 out]
      }
      frame True {
      }
    }
    "Camera Image Right" <- w168
  }
  n82 = while {
    tunnel: [w190] -> _
    tunnel: w59 -> [w184]
    tunnel: w58 -> [w181]
    i -> [w190]
    stop <- FALSE stop-if-true
    n83 = call <vilib>:"WPI_DashboardRetrieveStatusInfo.vi"("Binding Refnum"=w184, "Window Mode Notifier"=w181, "TCP Cnx"="TCP") -> ("Power and Errors"=w185:T21, "Robot Metrics"=w188:T22, "Status Info"=w189:T23, "Control Info"=w186:T24, "Robot Mode"=w183:T4, "Process?"=w187:bool)  [unwired: 3 in]
    "Mode" <- w183
    n84 = case shown="True" w187 {
      tunnel: w189 -> [_ w273]
      tunnel: w188 -> [_ w272]
      tunnel: w186 -> [_ w271]
      tunnel: w185 -> [_ w270]
      tunnel: w183 -> [_ _]
      frame False {
        n85 = Wait (ms)(milliseconds to wait=u32 20) -> ()  [unwired: 1 out]
      }
      frame True {
        # "swap motors to match\ncharts and include battery"
        n86 = Unbundle By Name(w271) -> ("Joystick Values"=w261:T25)  [unwired: 1 out]
        n87 = Unbundle By Name(w272) -> ()  [unwired: 1 out]
        n88 = Unbundle By Name(w270) -> ("Robot IP"=→"Robot IP":string)
        n89 = Unbundle By Name(w273) -> ("Battery V"=→"Battery Meter":dbl)  [unwired: 1 out]
        n90 = call "NET_Auto_Route.vi"("Read(F) Write(T)"=TRUE, "Route In"="Auto Route") -> ()  [unwired: 9 in, 1 out]
        n91 = Unbundle("H Values") -> (w245:dbl, w246:dbl)
        "H Max" <- w245
        "H Min" <- w246
        n92 = Unbundle("S Values") -> (w243:dbl, w244:dbl)
        "S Max" <- w243
        "S Min" <- w244
        n93 = Unbundle("V Values") -> (w241:dbl, w242:dbl)
        "V Max" <- w241
        "V Min" <- w242
        n94 = local read "Right Max"() -> (w214:dbl)
        n95 = local read "Left Max"() -> (w213:dbl)
        n96 = call "NET_Compressor.vi"("Read(F) Write(T)"=FALSE) -> ("Compressor Out"=w239:T26)  [unwired: 10 in]
        n97 = call "NET_Gear.vi"("Read(F) Write(T)"=FALSE) -> ("High Gear Out"=w233:bool)  [unwired: 10 in]
        "High Gear" <- w233
        n98 = call "NET_Drive_Cluster.vi"("Read(F) Write(T)"=FALSE) -> ("CMD_DriveCluster Out"=w230:T27)  [unwired: 10 in]
        n99 = call "NET_DriveRPM.vi"("Read(F) Write(T)"=FALSE) -> ("Right RPM Out"=w216:dbl, "Left RPM Out"=w215:dbl)  [unwired: 9 in]
        "Left" <- w215
        "Right" <- w216
        n100 = Unbundle By Name(w239) -> ("Compressor Running"=→"Comp. Running":bool, "Compressor Enabled"=→"Comp. Enabled":bool)
        n101 = Unbundle By Name(w230) -> ("Drive_Mode"=→"Drive Mode":T28, "Follow Cubes"=→"Cube":bool, "Lock Angle"=→"Lock Angle":bool, "Follow Road"=→"Road Nav":bool, "VBus.Turbo"=→"Turbo Enabled":bool)
        n102 = Greater?(x=w216, y=w214) -> (0:w218:bool)
        n103 = Not(x=w233) -> (.not. x?=→"Low Gear":bool)
        n104 = Greater?(x=w215, y=w213) -> (0:w217:bool)
        n105 = call "NET_Cube_HSV.vi"("H In Min"=w246, "H In Max"=w245, "S In Min"=w244, "S In Max"=w243, "V In Min"=w242, "V In Max"=w241, "Read(F) Write(T)"=TRUE) -> ()  [unwired: 15 in, 6 out]
        n106 = case shown="True" "Reset Max RPM" {
          tunnel: [w277 0] -> w220
          tunnel: [w275 0] -> w219
          tunnel: w218 -> [w279 _]
          tunnel: w217 -> [w278 _]
          tunnel: w216 -> [w276 _]
          tunnel: w215 -> [w274 _]
          frame False {
            n107 = case shown="False" w279 {
              tunnel: [w282 w283] -> w277
              tunnel: w276 -> [_ w283]
              frame False {
                n108 = local read "Right Max"() -> (w282:dbl)
              }
              frame True {
              }
            }
            n109 = case shown="False" w278 {
              tunnel: [w280 w281] -> w275
              tunnel: w274 -> [_ w281]
              frame False {
                n110 = local read "Left Max"() -> (w280:dbl)
              }
              frame True {
              }
            }
          }
          frame True {
          }
        }
        "Left Max" <- w219
        "Right Max" <- w220
        n111 = call-poly <vilib>:"NT Read Value.vi"("Name"="RobotDrive Motors") -> ("Numeric Array"=w251:dbl[])  [unwired: 9 in, 1 out]
        n112 = Index Array(array=w251, index #1=1, index #4=0) -> (element #1=w265:dbl, element #2=w266:dbl, element #3=w264:dbl, element #4=w269:dbl)  [unwired: 2 in]
        n113 = Index Array(array=w261) -> (element #1=w260:T32, element #2=w256:T32)  [unwired: 2 in]
        n114 = call "Prepare Joystick Data for Displays.vi"("Joystick Values"=w256) -> ("Buttons"=→"JS2 Buttons":T33, "Z Axis"=→"JS2 Z":dbl, "Cartesian Data"=→"JS2 Graph":cluster{"X axis":dbl, "X axis":dbl}[])  [unwired: 8 in]
        n115 = call "Prepare Joystick Data for Displays.vi"("Joystick Values"=w260) -> ("Buttons"=→"JS1 Buttons":T33, "Z Axis"=→"JS1 Z":dbl, "Cartesian Data"=→"JS1 Graph":cluster{"X axis":dbl, "X axis":dbl}[])  [unwired: 8 in]
        n116 = Bundle("Numeric"=w264, "Numeric"=w265) -> (→"MotorChart R" →"MotorSliders R":cluster{"Numeric":dbl, "Numeric":dbl})  [unwired: 1 in]
        n117 = Bundle("Numeric"=w266, "Numeric"=w269) -> (→"MotorChart L" →"MotorSliders L":cluster{"Numeric":dbl, "Numeric":dbl})  [unwired: 1 in]
        n118 = Bundle By Name(cluster=T20 {"High Gear Max"=0.0, "High Gear Min"=0.0, "Low Gear Max"=0.0, "Low Gear Min"=0.0} ("Cluster"), "High Gear Max"="High Gear Sen Max", "High Gear Min"="High Gear Sen Min", "Low Gear Min"="Low Gear Sen Min", "Low Gear Max"="Low Gear Sen Max") -> (w203:T20)
        n119 = call "NET_Limit_Switches.vi"("Read(F) Write(T)"=FALSE) -> ("Switches Out"=w211:T34)  [unwired: 10 in]
        n120 = call "NET_System_States.vi"("Read(F) Write(T)"=FALSE) -> ("Lift State Out"=→"Lift State":T6, "Claw Rotation State Out"=→"Claw Rotation State":T7, "Arm State Out"=→"Arm State":T8)  [unwired: 8 in]
        n121 = Unbundle By Name(w211) -> ("Cube"=→"Cube":bool, "Top Arm"=→"Top Arm":bool, "Top Lift"=→"Top Lift":bool, "Top Claw"=→"Top Claw":bool, "Bottom Arm"=→"Bottom Arm":bool, "Bottom Lift"=→"Bottom Lift":bool, "Bottom Claw"=→"Bottom Claw":bool)
        n122 = call "NET_Sensitivity.vi"("Read(F) Write(T)"=TRUE, "Sen In"=w203) -> ()  [unwired: 9 in, 1 out]
      }
    }
  }
  n123 = Index Array(array=w74) -> (element=w72:refnum<vi>)  [unwired: 1 in]
  n124 = control-ref of="Test Tree"() -> (w75:refnum<vi>)
  n125 = while {
    tunnel: [w295] -> _
    tunnel: w75 -> [w294]
    tunnel: w71 -> [w293]
    tunnel: w70 -> [w292]
    tunnel: w69 -> [_]
    tunnel: w65 -> [w291]
    tunnel: w53 -> [w290]
    tunnel: w52 -> [w289]
    shift-right: [w288] -> _
    shift-left: _ -> [w287]
    tunnel: w48 -> [w286]
    i -> [w295]
    stop <- FALSE stop-if-true
    n126 = event shown="[0] Timeout" {
      selector: w292 -> [_ _ _ _ _ _ _ _ _ _ _ _ _ _ _ _ _ _ _ _ _]
      dyn-events: [_ _ _ _ _ _ _ _ _ _ _ _ _ _ _ _ w555 _ _ _ _] -> _
      timeout: u32 60 ("milliseconds to wait") -> [_ _ _ _ _ _ _ _ _ _ _ _ _ _ _ _ _ _ _ _ _]
      tunnel: w294 -> [w307 _ _ _ _ _ _ _ _ _ _ _ _ _ _ _ _ _ _ _ _]
      tunnel: "Test Tree" -> [_ _ _ _ _ _ _ _ _ _ _ w522 w530 w532 w536 w544 _ _ _ _ _]
      tunnel: w293 -> [_ _ _ _ _ _ _ _ _ _ _ _ _ _ _ _ w557 _ w575 _ _]
      tunnel: w291 -> [_ _ _ _ _ _ _ _ _ _ _ _ _ _ _ _ w553 _ _ _ _]
      tunnel: w290 -> [_ _ _ _ _ _ _ _ _ _ _ _ _ _ _ _ w551 _ _ _ _]
      tunnel: w289 -> [w302 _ _ _ _ _ w473 _ _ _ _ _ _ _ _ _ _ _ _ _ _]
      tunnel: [w301 w350 w452 w457 w466 w470 w471 w480 w490 w497 w509 w521 w528 w531 w535 w543 w550 w570 w572 w576 w589] -> w288
      tunnel: w287 -> [w301 w350 w452 w457 w466 w470 w471 _ _ w497 w509 w521 w528 w531 w535 w543 w550 w570 w572 w576 w589]
      tunnel: w286 -> [w299 _ _ _ _ _ _ _ _ _ _ _ _ _ _ _ _ _ _ _ _]
      event Timeout {
        n127 = event-data() -> ()  [unwired: 1 in, 1 out]
        n128 = local read "Mode"() -> (w304:T4)
        n129 = case shown="\"Variables\"" "Dashboard Tab" {
          tunnel: w307 -> [_ w323 _ _]
          tunnel: "TestMode/Automatic/" ("Name Pattern") -> [_ w322 _ _]
          tunnel: T35 [{"Operation"=enum."Clear", "Color Box"=14013909}, {"Operation"=enum."Clear", "Color Box"=14013909}, {"Operation"=enum."Clear", "Color Box"=14013909}, {"Operation"=enum."Clear", "Color Box"=14013909}, {"Operation"=enum."Update", "Color Box"=14013909}, {"Operation"=enum."Update", "Color Box"=16777215}, {"Operation"=enum."Clear", "Color Box"=14013909}, {"Operation"=enum."Clear", "Color Box"=14013909}, {"Operation"=enum."Clear", "Color Box"=14013909}] -> [_ w315 _ w343]
          tunnel: w304 -> [_ w314 _ w342]
          tunnel: u32[] [15790320, 15790320, 15790320, 15790320, 16777215, 16777215, 15790320, 15790320, 15790320] -> [_ _ _ w348]
          tunnel: w302 -> [_ _ _ w336]
          tunnel: w299 -> [w309 _ _ _]
          frame "Auto", Default {
            n130 = call <vilib>:"WPI_DashboardUpdateNames.vi"("Controls on Tab"=w309) -> ()  [unwired: 11 in]
          }
          frame "Test" {
            w321 = -2 ("Active Item:Row Number")
            n131 = Index Array(array=w315, index=w314) -> (element=w316:T38)
            n132 = Unbundle(w316) -> ("Operation"=w317:enum16{"Update", "Clear"}, "Color Box"=w318:u32)
            n133 = call <vilib>:"NT Read String.vi"("Name"="TestMode/TestName") -> ("String"=w312:string)  [unwired: 9 in, 1 out]
            n134 = call <vilib>:"NT Read and Format Entries as Tree.vi"("Operation"=w317, "Name Pattern"=w322, "Tree Refnum"=w323) -> ()  [unwired: 7 in, 2 out]
            n135 = case shown="\"\"" w312 {
              tunnel: "TestMode/TestProgress" ("Name") -> [w325 _]
              tunnel: "TestMode/TestProgressText" ("Name") -> [w324 _]
              frame Default {
                n136 = call <vilib>:"NT Read Number.vi"("Name"=w325) -> ("Numeric"=w326:dbl)  [unwired: 9 in, 1 out]
                n137 = call <vilib>:"NT Read String.vi"("Name"=w324) -> ("String"=w327:string)  [unwired: 9 in, 1 out]
                n138 = Bundle("Numeric"=w326, "String"=w327) -> (→"Progress":cluster{"Numeric":dbl, "String":string})  [unwired: 1 in]
              }
              frame "" {
                n139 = property on="Progress" class="Clust (strict)"("Visible"=FALSE) -> ()  [unwired: 2 in, 2 out]
                n140 = local write "Test Name"(u16 0) -> ()
              }
            }
            n141 = property on="Test Tree" class="Tree (strict)"("Active Item Row Number"=w321, "ActiveColNum"=w321, "CellBG"=w318, "Active Item Row Number"=-1 ("Active Item:Row Number"), "CellBG"=u32 5789784 ("Color Box")) -> ()  [unwired: 2 in, 2 out]
          }
          frame "Variables" {
            w333 = string[] ["CameraPublisher", "Usage", "DB"]  # Items to initially close
            n142 = First Call?() -> (First Call?: T/F=w334:bool)
            n143 = control-ref of="Tree"() -> (w335:refnum<vi>)
            n144 = Select(t=w333, s=w334, f=string[] []) -> (s? t:f=w331:string[])
            n145 = call <vilib>:"NT Read and Format Entries as Tree.vi"("Tags to  Close"=w331, "Tree Refnum"=w335) -> ()  [unwired: 8 in, 2 out]
          }
          frame "Commands" {
            w344 = u32 5789784 ("Color Box")
            w345 = T39 {"Row"=-1, "Column"=-2} ("Active Cell:Active Cell")
            w347 = T39 {"Row"=-2, "Column"=-2} ("Active Cell:Active Cell")
            n146 = Index Array(array=w348, index=w342) -> (element=w346:u32)
            n147 = Index Array(array=w343, index=w342) -> (element=w341:T38)
            n148 = Unbundle(w341) -> ("Operation"=w340:enum16{"Update", "Clear"})  [unwired: 1 out]
            n149 = local read "Command Selection"() -> (w339:i32)
            n150 = property on="Command Selection" class="MCListbox (strict)"("ActiveCell"=w347, "CellBG"=w346, "ActiveCell"=w345, "CellBG"=w344) -> ()  [unwired: 2 in, 2 out]
            n151 = call <vilib>:"WPI_DashboardUpdate RPC Info.vi"("Operation"=w340) -> ("update"=w338:bool, "commands"=w337:string[][])  [unwired: 9 in]
            n152 = property on="Command Selection" class="MCListbox (strict)"("ItemNames"=w337) -> ()  [unwired: 2 in, 2 out]
            n153 = property on="Command Params" class="Tbl (strict)"("Active Cell"=w347, "Cell BG Color"=w346, "Active Cell"=w345, "Cell BG Color"=w344) -> ()  [unwired: 2 in, 2 out]
            n154 = call <vilib>:"WPI_DashboardUpdate Command Params.vi"("Update"=w338, "NewVal"=w339, "Commands"=w337, "Param Tbl"=w336) -> ()  [unwired: 7 in, 1 out]
          }
        }
        n155 = call <vilib>:"Connextion Info.vi"() -> ("Connected"=→"NT Connection":bool)  [unwired: 10 in, 1 out]
      }
      event "Test Tree": Value Change {
        # "Show appropriate\ncontrols"
        n156 = event-data() -> ("CtlRef"=w353:refnum<vi>, "NewVal"=w351:string)  [unwired: 1 in]
        n157 = call <vilib>:"WPI_UtilitiesGetTreeIOName.vi"("NewVal"=w351, "TreeControl in"=w353) -> ("I/O Name"=w354:string)  [unwired: 9 in]
        n158 = case shown="\"Camera\"" w354 {
          selector: w354 -> [_ w361 _ w383 w392 _]
          tunnel: w351 -> [_ _ w380 w382 _ w399]
          tunnel: cluster{string[]}[] [{["640x480", "320x240", "160x120"]}, {["Auto", "Fixed indoor", "Fixed outdoor 1", "Fixed outdoor 2", "Fixed fluorescent 1", "Fixed fluorescent 2", "Hold current"]}, {["Auto", "Flicker-free 50 Hz", "Flicker-free 60 Hz", "Hold current"]}, {["None", "Prioritize frame rate", "Prioritize image quality"]}, {["Monochrome", "Color"]}] -> [_ _ _ _ _ w398]
          frame Default {
            w356 = FALSE ("Visible")
            w355 = FALSE ("Visible")
            n159 = property on="Motor" class="Clust (strict)"("Visible"=w355) -> ()  [unwired: 2 in, 2 out]
            n160 = property on="Test Ring" class="Ring (strict)"("Visible"=w355) -> ()  [unwired: 2 in, 2 out]
            n161 = property on="Rev/Fwd" class="Clust (strict)"("Visible"=w356) -> ()  [unwired: 2 in, 2 out]
            n162 = property on="On/Off" class="Bool (strict)"("Visible"=w356) -> ()  [unwired: 2 in, 2 out]
            n163 = property on="Test Slider" class="Slide (strict)"("Visible"=w356) -> ()  [unwired: 2 in, 2 out]
          }
          frame "Analog Out", "Motor", "PWM" {
            w362 = FALSE ("Visible")
            n164 = case shown="\"Analog Out\"" w361 {
              tunnel: [1.0 ("Value") -1.0 ("Value") 0.0 ("Value")] -> w360
              tunnel: [255.0 ("Value") 1.0 ("Value") 5.0 ("Value")] -> w359
              tunnel: [128.0 ("Value") 0.0 ("Value") 0.0 ("Value")] -> w358
              tunnel: [64.0 ("Value") 0.5 ("Value") 1.0 ("Value")] -> w357
              frame "PWM" {
              }
              frame "Motor", Default {
              }
              frame "Analog Out" {
              }
            }
            n165 = property on="Motor" class="Clust (strict)"("Visible"=TRUE) -> ()  [unwired: 2 in, 2 out]
            n166 = property on="Value" class="Slide (strict)"("Value"=w358, "Scale.Minimum"=w360, "Scale.Maximum"=w359, "Scale.Increment"=w357) -> ()  [unwired: 2 in, 2 out]
            n167 = property on="On/Off" class="Bool (strict)"("Visible"=w362) -> ()  [unwired: 2 in, 2 out]
            n168 = property on="Test Slider" class="Slide (strict)"("Visible"=w362) -> ()  [unwired: 2 in, 2 out]
            n169 = property on="Test Ring" class="Ring (strict)"("Visible"=w362) -> ()  [unwired: 2 in, 2 out]
            n170 = property on="Rev/Fwd" class="Clust (strict)"("Visible"=w362) -> ()  [unwired: 2 in, 2 out]
          }
          frame "Servo" {
            w378 = FALSE ("Visible")
            n171 = call <vilib>:"NT Read Number.vi"("Name"=w380) -> ("Numeric"=w379:dbl)  [unwired: 9 in, 1 out]
            n172 = property on="Test Slider" class="Slide (strict)"("Visible"=TRUE, "Scale.Maximum"=170.0 ("Scale.Range:Maximum")) -> ()  [unwired: 2 in, 2 out]
            n173 = local write "Test Slider"(w379) -> ()
            n174 = property on="Motor" class="Clust (strict)"("Visible"=w378) -> ()  [unwired: 2 in, 2 out]
            n175 = property on="Rev/Fwd" class="Clust (strict)"("Visible"=w378) -> ()  [unwired: 2 in, 2 out]
            n176 = property on="On/Off" class="Bool (strict)"("Visible"=w378) -> ()  [unwired: 2 in, 2 out]
            n177 = property on="Test Ring" class="Ring (strict)"("Visible"=w378) -> ()  [unwired: 2 in, 2 out]
          }
          frame "Relay", "Solenoid" {
            w381 = FALSE ("Visible")
            n178 = property on="Motor" class="Clust (strict)"("Visible"=w381) -> ()  [unwired: 2 in, 2 out]
            n179 = property on="Test Slider" class="Slide (strict)"("Visible"=w381) -> ()  [unwired: 2 in, 2 out]
            n180 = Search and Replace String(input string=w382, search string="/Value  **", replace string="/Direction") -> (result string=w388:string)  [unwired: 5 in, 3 out]
            n181 = property on="Test Ring" class="Ring (strict)"("Visible"=w381) -> ()  [unwired: 2 in, 2 out]
            n182 = call <vilib>:"NT Read String.vi"("Name"=w388) -> ("String"=w386:string)  [unwired: 9 in, 1 out]
            n183 = Equal?(x="Both directions", y=w386) -> (x = y?=w384:bool)
            n184 = Not(x=w384) -> (.not. x?=w385:bool)
            n185 = property on="Rev/Fwd" class="Clust (strict)"("Visible"=w384) -> ()  [unwired: 2 in, 2 out]
            n186 = property on="On/Off" class="Bool (strict)"("Visible"=w385, "Caption.Text"=w383) -> ()  [unwired: 2 in, 2 out]
          }
          frame "Compressor", "Digital Out" {
            w391 = FALSE ("Visible")
            # "Get direction and finish"
            n187 = property on="Motor" class="Clust (strict)"("Visible"=w391) -> ()  [unwired: 2 in, 2 out]
            n188 = property on="Test Slider" class="Slide (strict)"("Visible"=w391) -> ()  [unwired: 2 in, 2 out]
            n189 = property on="Test Ring" class="Ring (strict)"("Visible"=w391) -> ()  [unwired: 2 in, 2 out]
            n190 = property on="On/Off" class="Bool (strict)"("Visible"=TRUE, "Caption.Text"=w392) -> ()  [unwired: 2 in, 2 out]
            n191 = property on="Rev/Fwd" class="Clust (strict)"("Visible"=FALSE) -> ()  [unwired: 2 in, 2 out]
          }
          frame "Camera" {
            n192 = call <vilib>:"Get Last Path Segment.vi"("String in"=w399) -> ("String out"=w400:string)  [unwired: 10 in]
            n193 = property on="On/Off" class="Bool (strict)"("Visible"=FALSE) -> ()  [unwired: 2 in, 2 out]
            n194 = property on="Motor" class="Clust (strict)"("Visible"=FALSE) -> ()  [unwired: 2 in, 2 out]
            n195 = property on="Rev/Fwd" class="Clust (strict)"("Visible"=FALSE) -> ()  [unwired: 2 in, 2 out]
            n196 = case shown="\"White Balance  **\"" w400 {
              tunnel: w399 -> [w406 w415 w424 w433 w442 _ w448]
              tunnel: w398 -> [w404 w412 w421 w430 w439 _ _]
              frame "Size  **" {
                n197 = Index Array(array=w404) -> (element=w403:cluster{string[]})  [unwired: 1 in]
                n198 = call <vilib>:"NT Read String.vi"("Name"=w406) -> ("String"=w405:string)  [unwired: 9 in, 1 out]
                n199 = Unbundle(w403) -> (w401:string[])
                n200 = Match First String(2:w401, 3:w405) -> (0:w402:i32)  [unwired: 1 out]
                n201 = property on="Test Ring" class="Ring (strict)"("Value"=w402, "Strings []"=w401) -> ()  [unwired: 2 in, 2 out]
                n202 = property on="Test Ring" class="Ring (strict)"("Visible"=TRUE) -> ()  [unwired: 2 in, 2 out]
                n203 = property on="Test Slider" class="Slide (strict)"("Visible"=FALSE) -> ()  [unwired: 2 in, 2 out]
              }
              frame "White Balance  **" {
                n204 = Index Array(array=w412, index=1) -> (element=w413:cluster{string[]})
                n205 = call <vilib>:"NT Read String.vi"("Name"=w415) -> ("String"=w414:string)  [unwired: 9 in, 1 out]
                n206 = Unbundle(w413) -> (w410:string[])
                n207 = Match First String(2:w410, 3:w414) -> (0:w409:i32)  [unwired: 1 out]
                n208 = property on="Test Ring" class="Ring (strict)"("Value"=w409, "Strings []"=w410) -> ()  [unwired: 2 in, 2 out]
                n209 = property on="Test Ring" class="Ring (strict)"("Visible"=TRUE) -> ()  [unwired: 2 in, 2 out]
                n210 = property on="Test Slider" class="Slide (strict)"("Visible"=FALSE) -> ()  [unwired: 2 in, 2 out]
              }
              frame "Exposure  **" {
                n211 = Index Array(array=w421, index=2) -> (element=w422:cluster{string[]})
                n212 = call <vilib>:"NT Read String.vi"("Name"=w424) -> ("String"=w423:string)  [unwired: 9 in, 1 out]
                n213 = Unbundle(w422) -> (w418:string[])
                n214 = Match First String(2:w418, 3:w423) -> (0:w419:i32)  [unwired: 1 out]
                n215 = property on="Test Ring" class="Ring (strict)"("Value"=w419, "Strings []"=w418) -> ()  [unwired: 2 in, 2 out]
                n216 = property on="Test Ring" class="Ring (strict)"("Visible"=TRUE) -> ()  [unwired: 2 in, 2 out]
                n217 = property on="Test Slider" class="Slide (strict)"("Visible"=FALSE) -> ()  [unwired: 2 in, 2 out]
              }
              frame "Exposure Priority  **" {
                n218 = Index Array(array=w430, index=3) -> (element=w431:cluster{string[]})
                n219 = call <vilib>:"NT Read String.vi"("Name"=w433) -> ("String"=w432:string)  [unwired: 9 in, 1 out]
                n220 = Unbundle(w431) -> (w427:string[])
                n221 = Match First String(2:w427, 3:w432) -> (0:w428:i32)  [unwired: 1 out]
                n222 = property on="Test Ring" class="Ring (strict)"("Value"=w428, "Strings []"=w427) -> ()  [unwired: 2 in, 2 out]
                n223 = property on="Test Ring" class="Ring (strict)"("Visible"=TRUE) -> ()  [unwired: 2 in, 2 out]
                n224 = property on="Test Slider" class="Slide (strict)"("Visible"=FALSE) -> ()  [unwired: 2 in, 2 out]
              }
              frame "Color Enable  **" {
                n225 = Index Array(array=w439, index=4) -> (element=w440:cluster{string[]})
                n226 = call <vilib>:"NT Read String.vi"("Name"=w442) -> ("String"=w441:string)  [unwired: 9 in, 1 out]
                n227 = Unbundle(w440) -> (w436:string[])
                n228 = Match First String(2:w436, 3:w441) -> (0:w437:i32)  [unwired: 1 out]
                n229 = property on="Test Ring" class="Ring (strict)"("Value"=w437, "Strings []"=w436) -> ()  [unwired: 2 in, 2 out]
                n230 = property on="Test Ring" class="Ring (strict)"("Visible"=TRUE) -> ()  [unwired: 2 in, 2 out]
                n231 = property on="Test Slider" class="Slide (strict)"("Visible"=FALSE) -> ()  [unwired: 2 in, 2 out]
              }
              frame Default {
                n232 = property on="Test Ring" class="Ring (strict)"("Visible"=FALSE) -> ()  [unwired: 2 in, 2 out]
                n233 = property on="Test Slider" class="Slide (strict)"("Visible"=FALSE) -> ()  [unwired: 2 in, 2 out]
              }
              frame "Brightness  **", "Color Level  **", "Compression  **", "FPS  **", "Sharpness  **" {
                n234 = call <vilib>:"NT Read Number.vi"("Name"=w448) -> ("Numeric"=w447:dbl)  [unwired: 9 in, 1 out]
                n235 = local write "Test Slider"(w447) -> ()
                n236 = property on="Test Slider" class="Slide (strict)"("Visible"=TRUE, "Scale.Maximum"=100.0 ("Scale.Range:Maximum")) -> ()  [unwired: 2 in, 2 out]
                n237 = property on="Test Ring" class="Ring (strict)"("Visible"=FALSE) -> ()  [unwired: 2 in, 2 out]
              }
            }
          }
        }
        n238 = property on="Progress" class="Clust (strict)"("Visible"=FALSE) -> ()  [unwired: 2 in, 2 out]
      }
      event "Test Name": Mouse Enter {
        # "Populate the ring with the list of tests"
        n239 = event-data() -> ()  [unwired: 1 in, 1 out]
        n240 = call <vilib>:"NT Read String Array.vi"("Name"="TestMode/TestList") -> ("String Array"=w456:string[])  [unwired: 9 in, 1 out]
        n241 = Build Array (concatenate)("Select the test to run...", w456) -> (w455:string[])
        n242 = property on="Test Name" class="Ring (strict)"("Strings []"=w455) -> ()  [unwired: 2 in, 2 out]
      }
      event "Test Name": Value Change {
        w458 = FALSE ("Visible")
        # "Tell the robot the test name to run"
        n243 = event-data() -> ("NewVal"=w462:u16)  [unwired: 1 in]
        n244 = property on="Test Name" class="Ring (strict)"() -> ("Strings []"=w463:string[])  [unwired: 2 in, 2 out]
        n245 = local write "Progress"(T11 {"Test Progress"=0, "Test Progress Text"=""} ("Progress")) -> ()
        n246 = Index Array(array=w463, index=w462) -> (element=w461:string)
        n247 = call <vilib>:"NT Write String.vi"("String"=w461, "Name"="TestMode/TestName") -> ()  [unwired: 9 in, 1 out]
        n248 = property on="Progress" class="Clust (strict)"("Visible"=TRUE) -> ()  [unwired: 2 in, 2 out]
        n249 = property on="Motor" class="Clust (strict)"("Visible"=w458) -> ()  [unwired: 2 in, 2 out]
        n250 = property on="Test Slider" class="Slide (strict)"("Visible"=w458) -> ()  [unwired: 2 in, 2 out]
        n251 = property on="On/Off" class="Bool (strict)"("Visible"=w458) -> ()  [unwired: 2 in, 2 out]
        n252 = property on="Rev/Fwd" class="Clust (strict)"("Visible"=w458) -> ()  [unwired: 2 in, 2 out]
        n253 = property on="Test Ring" class="Ring (strict)"("Visible"=w458) -> ()  [unwired: 2 in, 2 out]
      }
      event "Select Auto": Mouse Enter {
        # "Populate the combo box with the list of autonomous options"
        n254 = event-data() -> ()  [unwired: 1 in, 1 out]
        n255 = call <vilib>:"NT Read String Array.vi"("Name"="Auto List") -> ("String Array"=w465:string[])  [unwired: 9 in, 1 out]
        n256 = property on="Select Auto" class="CmbBox"("Strings[]"=w465) -> ()  [unwired: 2 in, 2 out]
      }
      event "Select Auto": Value Change {
        # "User modified the Auto Selection. Write to NT variable so robot knows."
        n257 = event-data() -> ("NewVal"=w468:string)  [unwired: 1 in]
        n258 = call <vilib>:"NT Write String.vi"("String"=w468, "Name"="Auto Selector") -> ()  [unwired: 9 in, 1 out]
      }
      event "Command Selection": Value Change {
        # "Get the params and show in table"
        n259 = event-data() -> ("NewVal"=w474:i32)  [unwired: 1 in]
        n260 = property on="Command Selection" class="MCListbox (strict)"() -> ("ItemNames"=w472:string[][])  [unwired: 2 in, 2 out]
        n261 = call <vilib>:"WPI_DashboardUpdate Command Params.vi"("NewVal"=w474, "Commands"=w472, "Param Tbl"=w473) -> ()  [unwired: 8 in, 1 out]
      }
      event "Execute Command": Value Change {
        # "Started one, Unique ID holds\nresponse"
        n262 = event-data() -> ()  [unwired: 1 in, 1 out]
        n263 = property on="Command Selection" class="MCListbox (strict)"() -> ("ItemNames"=w485:string[][])  [unwired: 2 in, 2 out]
        n264 = Index Array(array=w485, index (row)="Command Selection", index (col)=0) -> (element=w483:string)
        n265 = call <vilib>:"Invoke Commands.vi"("Command Params"="Command Params", "Function Name"=w483) -> ("Params"=w479:u8, "Started"=w478:bool)  [unwired: 7 in, 1 out]
        n266 = Array Subset(array="Command Params", length (row)=w479) -> (w480:string[][])  [unwired: 3 in]
        n267 = Select(t="Executing" ("Cmd Status"), s=w478, f="" ("Cmd Status")) -> (s? t:f=→"Cmd Status":string)
      }
      event "Command Selection": Double Click {
        n268 = event-data() -> ("Row"=w493:i32)  [unwired: 1 in]
        n269 = property on="Command Selection" class="MCListbox (strict)"() -> ("ItemNames"=w496:string[][])  [unwired: 2 in, 2 out]
        n270 = local read "Command Params"() -> (w492:string[][])
        n271 = Index Array(array=w496, index (row)=w493, index (col)=0) -> (element=w494:string)
        n272 = call <vilib>:"Invoke Commands.vi"("Command Params"=w492, "Function Name"=w494) -> ("Params"=w491:u8, "Started"=w486:bool)  [unwired: 7 in, 1 out]
        n273 = Array Subset(array=w492, length (row)=w491) -> (w490:string[][])  [unwired: 3 in]
        n274 = Select(t="Executing" ("Cmd Status"), s=w486, f="" ("Cmd Status")) -> (s? t:f=w487:string)
        n275 = local write "Cmd Status"(w487) -> ()
      }
      event "CheckList": Double Click {
        # "Shift clears all"
        # "Update symbols on the listbox"
        n276 = event-data() -> ("PlatMods.Shift"=w498:bool, "Row"=w500:i32)  [unwired: 1 in]
        n277 = case shown="True" w498 {
          tunnel: w500 -> [w504 _]
          tunnel: 1 -> [w503 _]
          frame False {
            n278 = property on="CheckList" class="LstBox (strict)"() -> ("Item Symbols"=w502:i32[])  [unwired: 2 in, 2 out]
            n279 = Replace Array Subset(array=w502, new element=w503, index=w504) -> (w501:i32[])
            n280 = property on="CheckList" class="LstBox (strict)"("Item Symbols"=w501) -> ()  [unwired: 2 in, 2 out]
          }
          frame True {
            w505 = 0 ("Top Row")
            n281 = property on="CheckList" class="LstBox (strict)"() -> ("Number of Rows"=w507:u32)  [unwired: 2 in, 2 out]
            n282 = Initialize Array(0, w507) -> (w506:i32[])
            n283 = property on="CheckList" class="LstBox (strict)"("Top Row"=w505, "Value"=w505, "Item Symbols"=w506) -> ()  [unwired: 2 in, 2 out]
          }
        }
      }
      event "CheckList": Key Down {
        # "Update symbols on the listbox\nLeft and right keys check and uncheck"
        n284 = event-data() -> ("VKey"=w511:T36)  [unwired: 1 in]
        n285 = case shown="\"Left\", \"Right\"" w511 {
          selector: w511 -> [w516 _]
          tunnel: eventvkey."Left" ("VKey") -> [w514 _]
          frame "Left", "Right" {
            n286 = Equal?(x=w514, y=w516) -> (x = y?=w515:bool)
            n287 = Select(t=0, s=w515, f=1) -> (s? t:f=w517:i32)
            n288 = property on="CheckList" class="LstBox (strict)"() -> ("Item Symbols"=w520:i32[])  [unwired: 2 in, 2 out]
            n289 = Replace Array Subset(array=w520, new element=w517, index="CheckList") -> (w519:i32[])
            n290 = property on="CheckList" class="LstBox (strict)"("Item Symbols"=w519) -> ()  [unwired: 2 in, 2 out]
          }
          frame Default {
          }
        }
      }
      event "Motor.Enable": Value Change {
        # "When the test mode otor enable helper is set, update that\ntree row item's value"
        n291 = event-data() -> ("NewVal"=w526:bool)  [unwired: 1 in]
        n292 = Unbundle("Motor") -> ("Value"=w525:dbl)  [unwired: 1 out]
        n293 = Select(t=w525, s=w526, f=0.0) -> (s? t:f=w523:dbl)
        n294 = call <vilib>:"NT Write Number.vi"("Numeric"=w523, "Name"=w522) -> ()  [unwired: 9 in, 1 out]
      }
      event "Test Slider": Value Change {
        # "When the test mode slider helper is set, update that\ntree row item's value"
        n295 = event-data() -> ("NewVal"=w529:dbl)  [unwired: 1 in]
        n296 = call <vilib>:"NT Write Number.vi"("Numeric"=w529, "Name"=w530) -> ()  [unwired: 9 in, 1 out]
      }
      event "On/Off": Value Change {
        # "When the test mode on/off helper value is set, update that\ntree row item's value"
        n297 = event-data() -> ("NewVal"=w534:bool)  [unwired: 1 in]
        n298 = Boolean To (0,1)(Boolean=w534) -> (0, 1=w533:i16)
        n299 = call <vilib>:"NT Write Number.vi"("Numeric"=w533, "Name"=w532) -> ()  [unwired: 9 in, 1 out]
      }
      event "Rev/Fwd": Value Change {
        # "When the test mode helper value for relays is set, update that\ntree row item's value"
        n300 = event-data() -> ("NewVal.Forward"=w542:bool, "NewVal.Reverse"=w541:bool)  [unwired: 1 in]
        n301 = Boolean To (0,1)(Boolean=w542) -> (0, 1=w538:i16)
        n302 = Boolean To (0,1)(Boolean=w541) -> (0, 1=w540:i16)
        n303 = Negate(x=w540) -> (-x=w539:i16)
        n304 = Add(x=w538, y=w539) -> (x+y=w537:i16)
        n305 = call <vilib>:"NT Write Number.vi"("Numeric"=w537, "Name"=w536) -> ()  [unwired: 9 in, 1 out]
      }
      event "Test Ring": Value Change {
        # "When a test mode helper value is selected from the ring,\nset the tree item's variable to the string value"
        n306 = event-data() -> ("NewVal"=w546:u16)  [unwired: 1 in]
        n307 = property on="Test Ring" class="Ring (strict)"() -> ("Strings []"=w547:string[])  [unwired: 2 in, 2 out]
        n308 = Index Array(array=w547, index=w546) -> (element=w545:string)
        n309 = call <vilib>:"NT Write String.vi"("String"=w545, "Name"=w544) -> ()  [unwired: 9 in, 1 out]
      }
      event "Rec Mode": Value Change {
        # "Update globals for recording mode and path to read log from.\nClear when logging and let NetworkTables set path for vision to\nuse."
        n310 = event-data() -> ("NewVal"=w558:enum32{"Stop", "Record", "Playback"})  [unwired: 1 in]
        n311 = global write "WPI_DashboardLogging Global.vi" "Logging Filename"(path "") -> ()
        n312 = global write "WPI_DashboardLogging Global.vi" "Recording"(w558) -> ()
        n313 = case shown="\"Playback\"" w558 {
          tunnel: w557 -> [_ w560 w569]
          tunnel: [_ _ w568] -> w555
          tunnel: [_ _ w567] -> _
          tunnel: w553 -> [_ _ w565]
          tunnel: cluster{i32, i32} {-250, 170} -> [_ _ w564]
          tunnel: [_ _ T37 {"Image Size"=TRUE, "Image Type"=TRUE, "Pixel Value"=TRUE, "ROI Information"=TRUE, "Zoom Factor"=FALSE} ("Image Information Shown:All Elements")] -> w548
          tunnel: [_ _ TRUE ("Zoom Factor")] -> w549
          tunnel: w551 -> [_ _ w561]
          frame Default {
          }
          frame "Stop", "Record" {
            # "Place Window too"
            n314 = invoke class="VI" method="FP.Close"(reference=w560) -> (reference out=w559:refnum<vi>)  [unwired: 2 in, 2 out]
            n315 = invoke class="VI" method="Abort VI"(reference=w559) -> ()  [unwired: 2 in, 3 out]
          }
          frame "Playback" {
            n316 = call "Open Playback Panel.vi"("Offset"=w564, "DB VI Ref"=w565, "Playback in"=w569) -> ("Playback out"=w566:refnum<vi>)  [unwired: 8 in]
            n317 = register-events(w566, w561) -> (reference out=w568:refnum<event-registration>, error out=w567:errorcluster)  [unwired: 2 in]
          }
        }
        n318 = property on="Camera Image Right" class="ImageControl"("Image Information Shown"=w548, "Image Information Visible"=w549) -> ()  [unwired: 2 in, 2 out]
        n319 = property on="Camera Image" class="ImageControl"("Image Information Shown"=w548, "Image Information Visible"=w549) -> ()  [unwired: 2 in, 2 out]
        n320 = call <vilib>:"WPI_DashboardNT Log FieldName Cache.vi"("Operation"=enum16{"Lookup/Add", "Index", "Clear"}."Clear") -> ()  [unwired: 8 in, 3 out]
      }
      event Panel Close {
        w571 = enum32{"Stop", "Record", "Playback"}."Stop" ("Rec Mode")
        # "Playback window has been closed, abort"
        n321 = event-data() -> ()  [unwired: 1 in, 4 out]
        n322 = local write "Rec Mode"(w571) -> ()
        n323 = global write "WPI_DashboardLogging Global.vi" "Recording"(w571) -> ()
      }
      event Panel Close {
        # "Abort playback window and ourself"
        n324 = event-data() -> ()  [unwired: 1 in, 4 out]
        n325 = invoke class="VI" method="FP.Close"(reference=w575) -> (reference out=w574:refnum<vi>)  [unwired: 2 in, 2 out]
        n326 = invoke class="VI" method="Abort VI"(reference=w574) -> (error out=w573:errorcluster)  [unwired: 2 in, 2 out]
        n327 = invoke class="VI" method="Abort VI"(error in=w573) -> ()  [unwired: 2 in, 3 out]
      }
      event User Event {
        n328 = event-data() -> ("IDs"=w582:cluster{"RPC field ID":u16, "Unique ID":u16}, "String"=w581:string)  [unwired: 1 in]
        n329 = Bundle("IDs"=w582, "String"=w581) -> (w580:T15)  [unwired: 1 in]
        n330 = call <vilib>:"Retrieve RPC Response.vi"("RPC Response"=w580) -> ("Output"=w578:string[][])  [unwired: 10 in]
        n331 = Build Array (concatenate)(w576, w578) -> (w577:string[][])
        n332 = local write "Command Params"(w577) -> ()
        n333 = local write "Cmd Status"("" ("Cmd Status")) -> ()
      }
      event "Tree": Double Click {
        n334 = event-data() -> ("PlatMods"=w588:T40, "Tag"=w585:string)  [unwired: 1 in]
        n335 = Unbundle(w588) -> ("Shift"=w587:bool)  [unwired: 4 out]
        n336 = String Subset(string=w585, length (rest)=1 ("length (rest)")) -> (substring=w584:string)  [unwired: 1 in]
        n337 = Not(x=w587) -> (.not. x?=w586:bool)
        n338 = case shown="\"/\"" w584 {
          tunnel: w585 -> [_ w591]
          tunnel: w586 -> [_ w590]
          frame Default {
          }
          frame "/" {
            n339 = call <vilib>:"NT Update Persistence.vi"("Persistence"=w590, "Name"=w591) -> ()  [unwired: 9 in, 1 out]
          }
        }
      }
    }
  }
  n340 = while {
    tunnel: w72 -> [w593]
    i -> [w596]
    stop <- FALSE stop-if-true
    n341 = Wait (ms)(milliseconds to wait=u32 100) -> ()  [unwired: 1 out]
    n342 = case shown="\"Playback\"" "Rec Mode" {
      tunnel: w596 -> [_ _ w611]
      tunnel: [u32 2829099 ("Base Color") u32 11141120 ("Target Color") w600] -> w592
      frame "Stop", Default {
        # "Reset the color, extra updates don't cost much"
      }
      frame "Record" {
      }
      frame "Playback" {
        # "Playback"
        n343 = Quotient & Remainder(x=w611, y=u32 50 ("milliseconds to wait")) -> (x-y*floor(x/y)=w607:u32)  [unwired: 1 out]
        n344 = Divide(x=w607, y=u32 50 ("milliseconds to wait")) -> (x/y=w604:dbl)
        n345 = Multiply(x=6.283185307179586, y=w604) -> (x*y=w609:dbl)
        n346 = Sine(x=w609) -> (sin(x)=w608:dbl)
        n347 = Absolute Value(x=w608) -> (abs(x)=w601:dbl)
        n348 = call "Interpolate RGB Color.vi"("Proportion"=w601, "Target Color"=u32 30976, "Base Color"=u32 2829099) -> ("Result Color"=w600:u32)  [unwired: 8 in]
      }
    }
    n349 = property class="Pane"(reference=w593, "PaneColor"=w592) -> ()  [unwired: 1 in, 2 out]
  }
  n350 = local write "Dashboard Tab"(T16."Test" ("Dashboard Tab")) -> ()
  n351 = property on="On/Off" class="Bool (strict)"("Visible"=w60) -> ()  [unwired: 2 in, 2 out]
  n352 = property on="Motor" class="Clust (strict)"("Visible"=w60) -> ()  [unwired: 2 in, 2 out]
  n353 = property on="Progress" class="Clust (strict)"("Visible"=w60) -> ()  [unwired: 2 in, 2 out]
  n354 = property on="Test Ring" class="Ring (strict)"("Visible"=w60) -> ()  [unwired: 2 in, 2 out]
  n355 = property on="Rev/Fwd" class="Clust (strict)"("Visible"=w60) -> ()  [unwired: 2 in, 2 out]
  n356 = property on="Handsome Hale" class="Pict"() -> ("Width"=w19:u32, "Height"=w20:u32)  [unwired: 2 in, 2 out]
  n357 = property on="Jeffery Junior" class="Pict"() -> ("Width"=w2:u32, "Height"=w1:u32)  [unwired: 2 in, 2 out]
  n358 = property on="Manipulator Mietus" class="Pict"() -> ("Width"=w22:u32, "Height"=w21:u32)  [unwired: 2 in, 2 out]
  n359 = local write "Command Selection"(u16 0 ("milliseconds to wait")) -> ()
  n360 = call <vilib>:"Read JPEG File.vi"("path to JPEG file"=path "Images/Joeseph.jpg" ("path to PNG file")) -> ("image data"=w12:T41)  [unwired: 8 in, 2 out]
  n361 = call <vilib>:"Read JPEG File.vi"("path to JPEG file"=path "Images/Baby.jpg" ("path to PNG file")) -> ("image data"=w9:T41)  [unwired: 8 in, 2 out]
  n362 = Unbundle By Name(w12) -> ("Rectangle.right"=w13:i16, "Rectangle.bottom"=w14:i16)
  n363 = Unbundle By Name(w9) -> ("Rectangle.right"=w8:i16, "Rectangle.bottom"=w7:i16)
  n364 = call <vilib>:"Read JPEG File.vi"("path to JPEG file"=path "Images/Amanda.jpg" ("path to PNG file")) -> ("image data"=w29:T41)  [unwired: 8 in, 2 out]
  n365 = Unbundle By Name(w29) -> ("Rectangle.right"=w28:i16, "Rectangle.bottom"=w27:i16)
  n366 = call <vilib>:"Draw Flattened Pixmap.vi"("image data"=w12) -> ("new picture"=→"Handsome Hale":picture)  [unwired: 8 in]
  n367 = call <vilib>:"Draw Flattened Pixmap.vi"("image data"=w9) -> ("new picture"=→"Jeffery Junior":picture)  [unwired: 8 in]
  n368 = Divide(x=w19, y=w13) -> (x/y=w15:dbl)
  n369 = Divide(x=w20, y=w14) -> (x/y=w16:dbl)
  n370 = Divide(x=w2, y=w8) -> (x/y=w6:dbl)
  n371 = Divide(x=w1, y=w7) -> (x/y=w5:dbl)
  n372 = call <vilib>:"Draw Flattened Pixmap.vi"("image data"=w29) -> ("new picture"=→"Manipulator Mietus":picture)  [unwired: 8 in]
  n373 = Divide(x=w22, y=w28) -> (x/y=w26:dbl)
  n374 = Divide(x=w21, y=w27) -> (x/y=w25:dbl)
  n375 = local write "Command Params"(string[][] [] ("Command Params")) -> ()
  n376 = Max & Min(x=w15, y=w16) -> (min(x,y)=w18:dbl)  [unwired: 1 out]
  n377 = Max & Min(x=w6, y=w5) -> (min(x,y)=w3:dbl)  [unwired: 1 out]
  n378 = global write "WPI_DashboardLogging Global.vi" "Recording"(w66) -> ()
  n379 = local write "Rec Mode"(w66) -> ()
  n380 = Max & Min(x=w26, y=w25) -> (min(x,y)=w23:dbl)  [unwired: 1 out]
  n381 = call <vilib>:"NT Write String.vi"("String"="Select Auto", "Name"="Auto Selector") -> ()  [unwired: 9 in, 1 out]
  n382 = property on="Handsome Hale" class="Pict"("ZoomFactor"=w18) -> ()  [unwired: 2 in, 2 out]
  n383 = property on="Jeffery Junior" class="Pict"("ZoomFactor"=w3) -> ()  [unwired: 2 in, 2 out]
  n384 = property on="Manipulator Mietus" class="Pict"("ZoomFactor"=w23) -> ()  [unwired: 2 in, 2 out]
  n385 = while {
    tunnel: u16 1741 ("timeout ms (25000)") -> [w613]
    stop <- FALSE stop-if-true
    n386 = TCP Create Listener(10:w613) -> (0:w612:errorcluster, 3:w614:refnum<k5>)  [unwired: 4 in, 1 out]
    n387 = case shown="No Error" w612 {
      selector: w612 -> [w616 _]
      tunnel: w614 -> [w617 _]
      frame No Error {
        n388 = while {
          tunnel: w617 -> [w620]
          tunnel: w616 -> [w619]
          stop <- FALSE stop-if-true
          n389 = TCP Wait On Listener(8:w619, 11:w620) -> (0:w621:errorcluster, 4:w622:refnum<k5>)  [unwired: 2 in, 3 out]
          n390 = local write "TCP"(w622) -> ()
          n391 = case shown="No Error" w621 {
            frame No Error {
            }
            frame Error {
              n392 = Wait (ms)(milliseconds to wait=u32 1000) -> ()  [unwired: 1 out]
            }
          }
        }
      }
      frame Error {
        n393 = Wait (ms)(milliseconds to wait=u32 1000) -> ()  [unwired: 1 out]
      }
    }
  }
